vi "Boolean Debounce.vi"(2 "Boolean in":bool, 3 "Default":bool) -> (0 "Boolean out":bool)   [LabVIEW 2012]
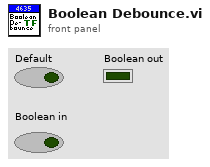
[diagram p1: front panel]
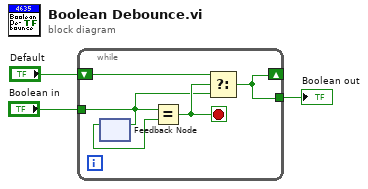
[diagram p0: block diagram]
diagram:
  n1 = while {
    shift-right: [w7] -> _
    shift-left: "Default" -> [w8]
    tunnel: [w7] -> w3
    tunnel: "Boolean in" -> [w4]
    stop <- w5 stop-if-true
    n2 = feedback-in #1(w4) -> ()
    n3 = feedback #1() -> (w6:bool)  [unwired: 1 in]
    n4 = Equal?(x=w4, y=w6) -> (x = y?=w5:bool)
    n5 = Select(t=w8, s=w5, f=w4) -> (s? t:f=w7:bool)
  }
  "Boolean out" <- w3
